vi "RegisterMatOrNumber_Array1D-4DPoint-I32.vi"(0 "Array in":T1[](array[typedef]), 11 "error in":errorcluster) -> (4 "Image":u8, 12 "Value":dbl, 13 "Mat":T2, 14 "AdressOrData":T1[](array[typedef]), 15 "error out":errorcluster)   [LabVIEW 2020, in "OpenLvVision_OpenCv.lvlib"]
doc: "Register mat or value for dll.\nNo malleable to breake vi inlining!"
uses:
  TypeDef/MatInfo.ctl
  TypeDef/LvDatatype.ctl
  OpenLvVision_OpenCv.lvlib
  TypeDef/Point/4D_PointI32.ctl
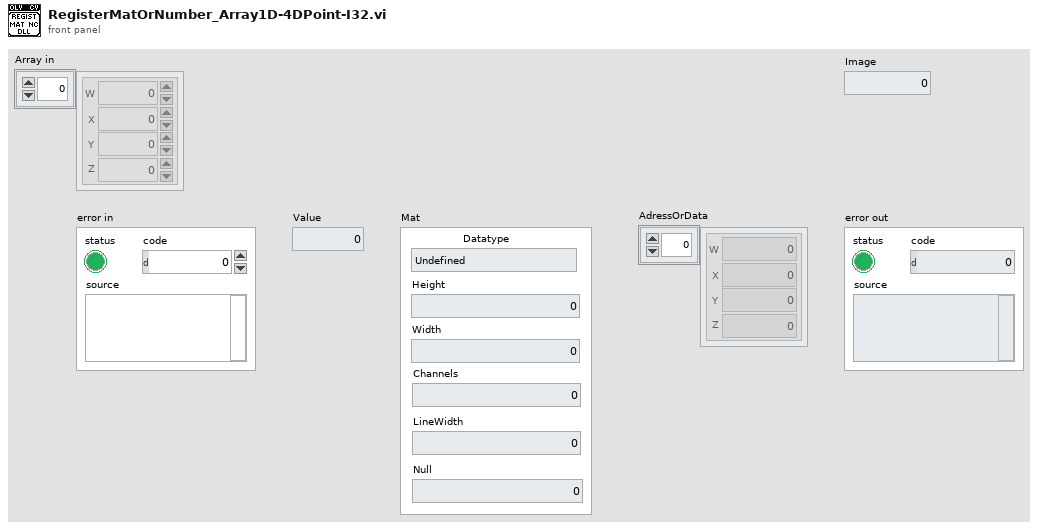
[diagram p1: front panel]
types:
  T1 = typedef "OpenLvVision_OpenCv.lvlib/4D_PointI32.ctl" = cluster{"W":i32, "X":i32, "Y":i32, "Z":i32}
  T2 = typedef "OpenLvVision_OpenCv.lvlib/MatInfo.ctl" = cluster{"Datatype":T3, "Height":i32, "Width":i32, "Channels":i32, "LineWidth":i32, "Null":u8}
  T3 = typedef "OpenLvVision_OpenCv.lvlib/LvDatatype.ctl" = enum32{"Undefined", "U8", "I8", "U16", "I16", "U32_Color", "I32", "U64_Color", "I64", "SGL", "DBL", "Complex SGL", "Complex DBL", "Array 1D U8", "Array 1D I8", "Array 1D U16", "Array 1D I16", "Array 1D U32_Color", "Array 1D I32", "Array 1D U64_Color", "Array 1D I64", "Array 1D SGL", "Array 1D DBL", "Array 1D Complex SGL", "Array 1D Complex DBL", "Array 2D U8", "Array 2D I8", "Array 2D U16", "Array 2D I16", "Array 2D U32", "Array 2D U32_Color", "Array 2D I32", "Array 2D U64", "Array 2D U64_Color", "Array 2D I64", "Array 2D SGL", "Array 2D DBL", "Array 2D Complex SGL", "Array 2D Complex DBL", "Image Mono U8", "Image Mono U16", "Image Mono I16", "Image Mono SGL", "Image Color U32", "Image Color U64", "ImageComplex Sgl", "Array1d_2dPointI32", "Array1d_2dPointSGL", "Array1d_2dPointDBL", "Array1d_3dPointI32", "Array1d_3dPointSGL", "Array1d_3dPointDBL", "Array1d_4dPointI32", "Array1d_4dPointSGL", "Array1d_4dPointDBL"}
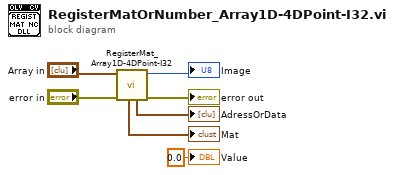
[diagram p0: block diagram]
diagram:
  n1 = call "RegisterMat_Array1D-4DPoint-I32.vi"("error in"="error in", "Array in"="Array in") -> ("error out"=→"error out":errorcluster, "Image"=→"Image":u8, "AdressOrData"=→"AdressOrData":T1[], "Mat"=→"Mat":T2)  [unwired: 6 in]
  "Value" <- 0.0 ("Value")
